vi "Read Supported Functions.vi"(8 "error in (no error)":errorcluster, 11 "Visa instrument in":refnum<class "Visa instrument.lvclass">) -> (0 "error out":errorcluster, 2 "Supported Functions":T1[](array[typedef])=[enum."Input"], 3 "Visa instrument out":refnum<class "Visa instrument.lvclass">)   [LabVIEW 2015, in "Visa instrument.lvclass"]
uses:
  Visa instrument.lvclass
  Mag Lab Hardware Function.ctl
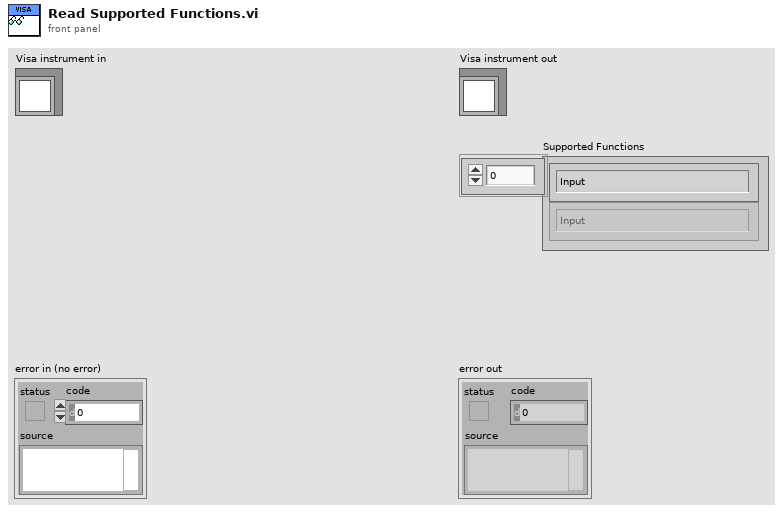
[diagram p1: front panel]
types:
  T1 = typedef "Mag Lab Hardware Function.ctl" = enum16{"Input", "Voltmeter", "Output", "Current source", "Digitizer", "Temperature controller"}
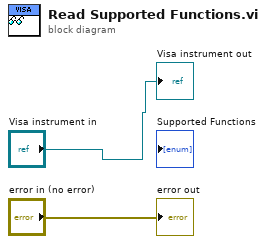
[diagram p0: block diagram]
diagram:
  "error out" <- "error in (no error)"
  "Visa instrument out" <- "Visa instrument in"
